vi "Read Channel Info.vi"(8 "error in (no error)":errorcluster, 11 "DAQmx Analog.lvclass in":refnum<class "DAQmx Analog.lvclass">) -> (0 "error out":errorcluster, 1 "Channel Units":string[](array[string]), 2 "Channel Names":string[](array[string]), 3 "DAQmx Analog.lvclass out":refnum<class "DAQmx Analog.lvclass">, 5 "#Channels":i32)   [LabVIEW 2009, in "DAQmx Analog.lvclass"]
doc: "(Dynamic) Return information about the readable data channels this object provides, e.g., the name of each data source and its unit."
uses:
  DAQmx Analog.lvclass
  Utility Classes/Readable/Readable.lvclass
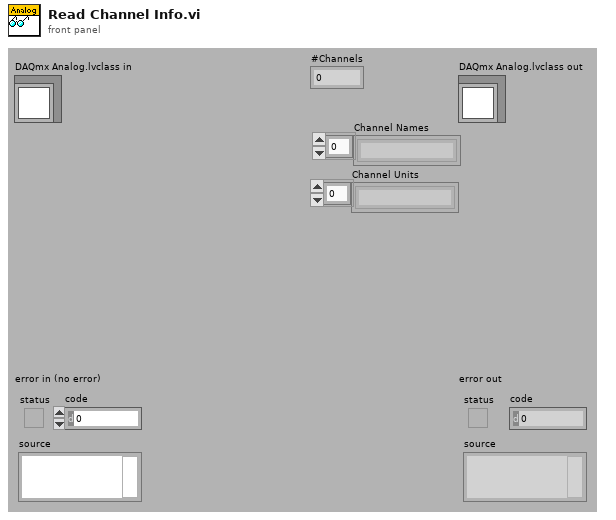
[diagram p1: front panel]
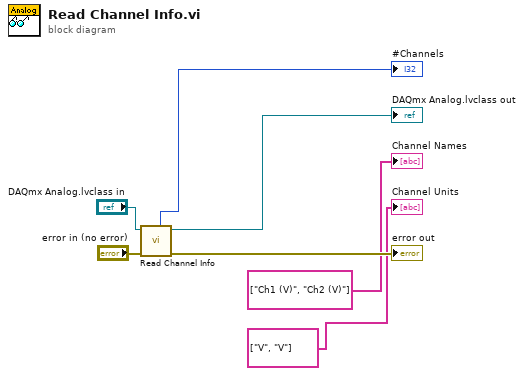
[diagram p0: block diagram]
diagram:
  n1 = call-parent "Read Channel Info.vi"("error in (no error)"="error in (no error)", "Readable.lvclass in"="DAQmx Analog.lvclass in") -> ("error out"=→"error out":errorcluster, "Readable.lvclass out"=→"DAQmx Analog.lvclass out":refnum<class "DAQmx Analog.lvclass">, "#Channels"=→"#Channels":i32)  [unwired: 5 in, 2 out]
  "Channel Units" <- string[] ["V", "V"] ("Channel Units")
  "Channel Names" <- string[] ["Ch1 (V)", "Ch2 (V)"] ("Channel Names")
